vi "SetAiScale.vi"(0 "Array":refnum<class "Sig_AI.lvclass">[](array[class]), 11 "error in (no error)":errorcluster) -> (4 "Array 2":refnum<class "Sig_AI.lvclass">[](array[class]), 15 "error out":errorcluster)   [LabVIEW 2019]
uses:
  Sig_AI_class/Sig_AI.lvclass
  TypeDef/SensorCalibrationData_Array.ctl
  TypeDef/SensorCalibrationData.ctl
  TypeDef/CalbrationPoint.ctl
  TypeDef/Channel Setting Array.ctl
  TypeDef/GUI Setting Channel.ctl
  TypeDef/Config_Scale.ctl
  Sig_AI_class/Sig_AI.lvclass/Sig_AI.ctl
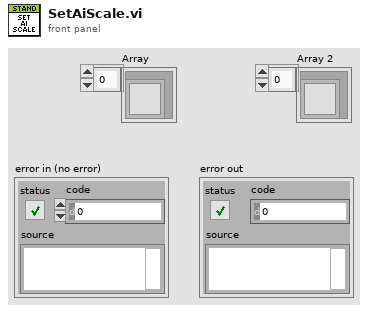
[diagram p1: front panel]
types:
  T1 = typedef "SensorCalibrationData_Array.ctl" = cluster{"SENSORS_ARR":T2[]}
  T2 = typedef "SensorCalibrationData.ctl" = cluster{"Name":string, "ID":u32, "Slope":dbl, "Intercept":dbl, "Calibration":T3[]}
  T3 = typedef "CalbrationPoint.ctl" = cluster{"RAW":dbl, "SCL":dbl}
  T4 = typedef "Channel Setting Array.ctl" = cluster{"Channels data":T5[]}
  T5 = typedef "GUI Setting Channel.ctl" = cluster{"Name":string, "SensorID":u32}
  T6 = typedef "Config_Scale.ctl" = cluster{"scale [EU/RAW]":dbl, "offset [EU]":dbl}
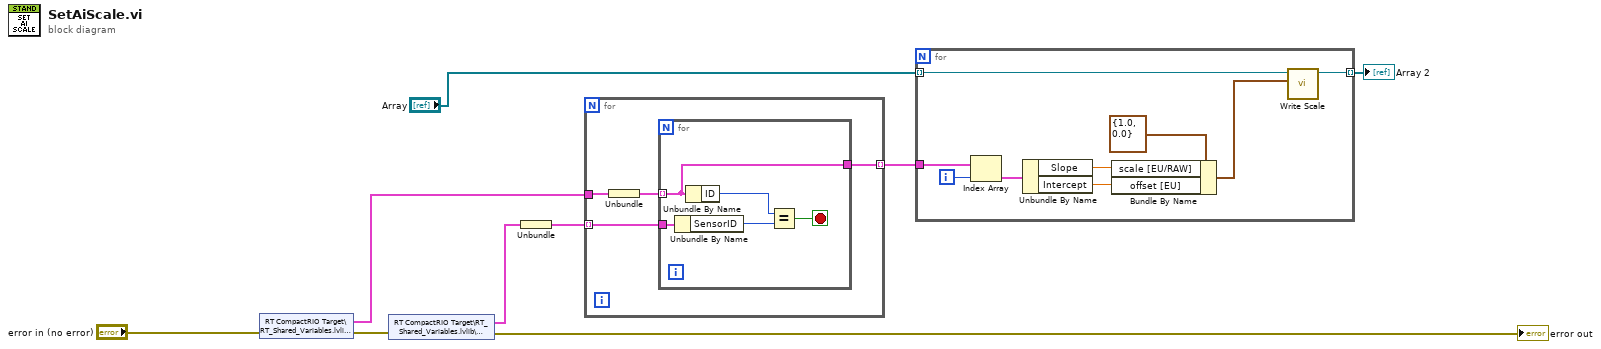
[diagram p0: block diagram]
diagram:
  n1 = shared-variable "RT CompactRIO Target\\RT_Shared_Variables.lvlib\\SENSORS"(error in="error in (no error)") -> (w4:T1, error out=w7:errorcluster)
  n2 = shared-variable "RT CompactRIO Target\\RT_Shared_Variables.lvlib\\CHANNELS"(error in=w7) -> (w6:T4, error out=→"error out":errorcluster)
  n3 = Unbundle(w6) -> ("Channels data"=w5:T5[])
  n4 = for {
    tunnel: w5 -> [w13] mode=indexing
    tunnel: w4 -> [w12]
    tunnel: [w10] -> w3 mode=indexing
    n5 = Unbundle(w12) -> ("SENSORS_ARR"=w11:T2[])
    n6 = for {
      tunnel: w13 -> [w18]
      tunnel: w11 -> [w14] mode=indexing
      tunnel: [w14] -> w10
      stop <- w15 stop-if-true
      n7 = Unbundle By Name(w18) -> ("SensorID"=w17:u32)
      n8 = Unbundle By Name(w14) -> ("ID"=w16:u32)
      n9 = Equal?(x=w16, y=w17) -> (x = y?=w15:bool)
    }
  }
  n10 = for {
    tunnel: [w23] -> w1 mode=indexing
    tunnel: "Array" -> [w24] mode=indexing
    tunnel: w3 -> [w27]
    i -> [w26]
    n11 = Index Array(array=w27, index=w26) -> (element=w25:T2)
    n12 = Unbundle By Name(w25) -> ("Slope"=w20:dbl, "Intercept"=w19:dbl)
    n13 = Bundle By Name(cluster=T6 {"scale [EU/RAW]"=1.0, "offset [EU]"=0.0} ("ConfigScale"), "scale [EU/RAW]"=w20, "offset [EU]"=w19) -> (w21:T6)
    n14 = call "Write Scale.vi"("ConfigScale"=w21, "Sig_AI in"=w24) -> ("Sig_AI out"=w23:refnum<class "Sig_AI.lvclass">)  [unwired: 9 in]
  }
  "Array 2" <- w1
